vi "Boiler.vi"() -> ()   [LabVIEW 2025]
uses:
  Controls/Boiler Controls.ctl
  Controls/Boiler Simulation Controls.ctl
  Controls/Boiler Status Indicators.ctl
  Controls/States.ctl
panel:
  in  "stop":bool
  out "Boiler Status Indicators":T1 {"Time Count" format="%.2g"}
  in  "Boiler Simulation Controls":T2 {"Flame Sensor Value (%)" min=0.0 max=100.0 scale=0.0..100.0}
  in  "Boiler Controls":T3 {"Fuel Valve Position" min=0.0 max=100.0 scale=0.0..100.0 scale format="%.2f"}
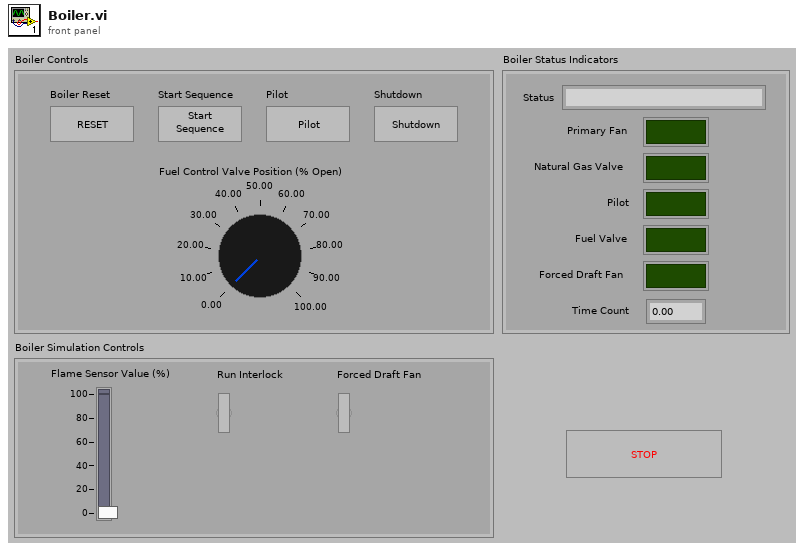
[diagram p1: front panel]
types:
  T1 = typedef "Boiler Status Indicators.ctl" = cluster{"Status":string, "Primary Fan":bool, "Natural Gas Valve":bool, "Pilot":bool, "Fuel Valve":bool, "Forced Draft Fan":bool, "Time Count":dbl}
  T2 = typedef "Boiler Simulation Controls.ctl" = cluster{"Flame Sensor Value (%)":dbl, "Run Interlock":bool, "Forced Draft Fan":bool}
  T3 = typedef "Boiler Controls.ctl" = cluster{"Boiler Reset":bool, "Start Sequence":bool, "Pilot":bool, "Shutdown":bool, "Fuel Valve Position":dbl}
  T4 = typedef "States.ctl" = enum16{"Initialization", "Lockout", "Ready", "Pre-Purge Start", "Pre-Purge Ongoing", "Pre-Purge Complete", "Wait Pilot", "Pilot-On", "Boiler Ready", "Fan On", "Boiler Running", "Shutdown Purge Start", "Shutdown Purge Ongoing", "Shutdown Purge Complete"}
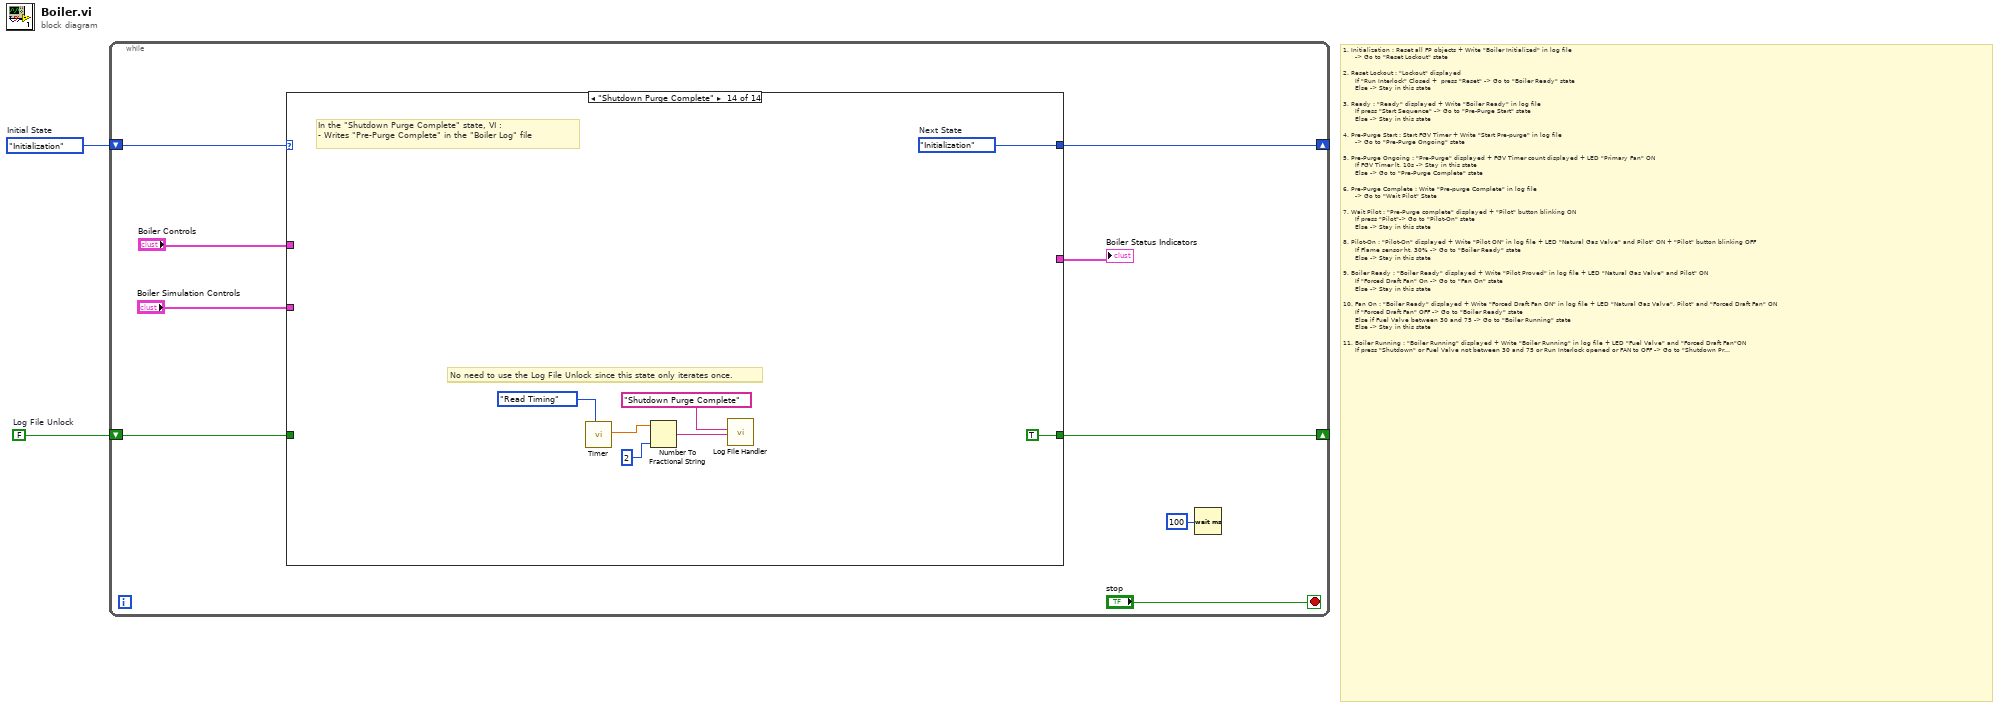
[diagram p0: block diagram]
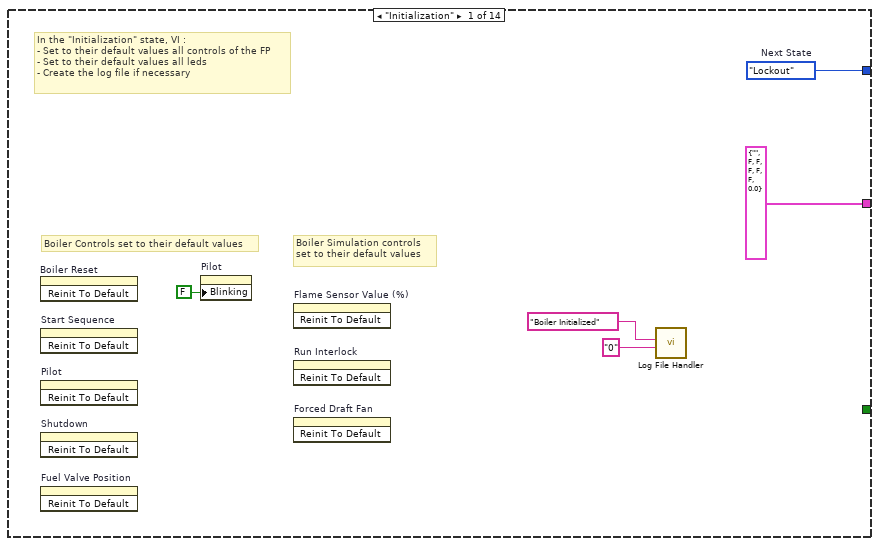
[diagram p2: hidden frame]
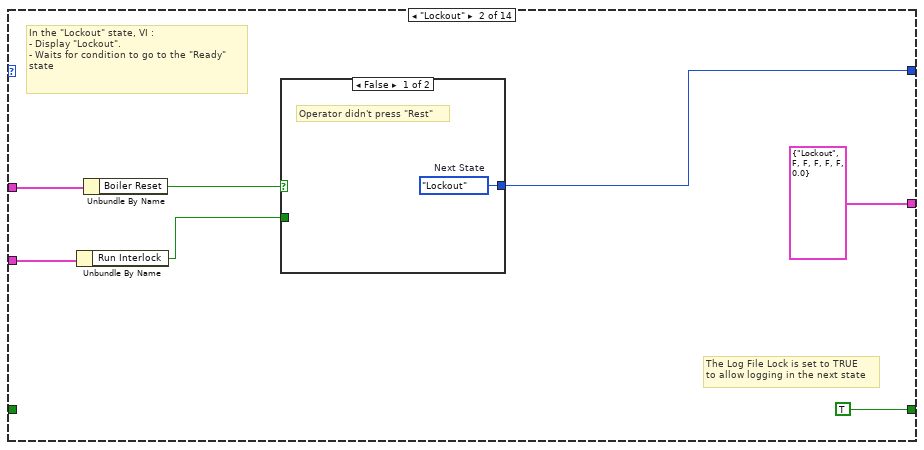
[diagram p3: hidden frame]
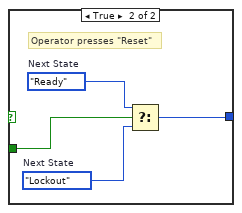
[diagram p4: hidden frame]
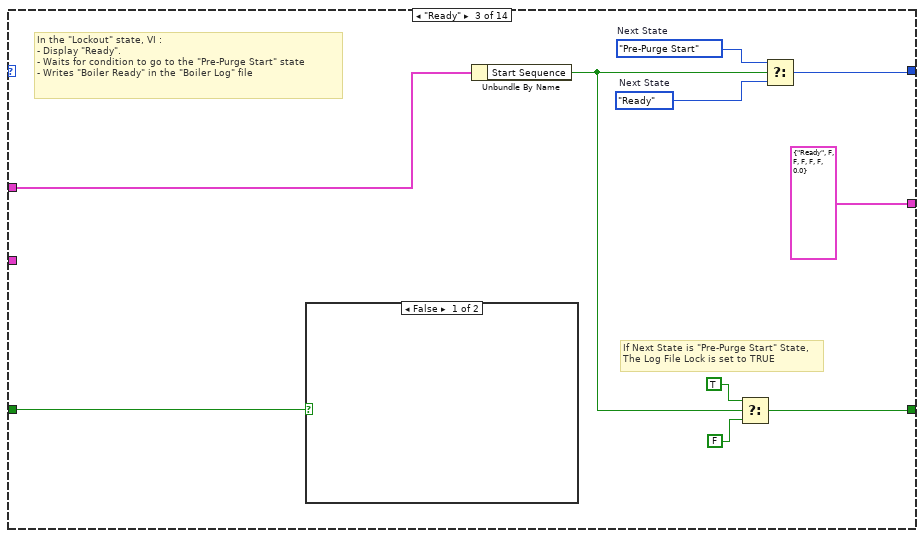
[diagram p5: hidden frame]
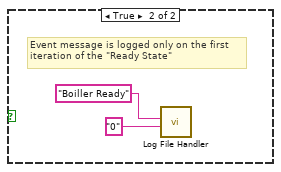
[diagram p6: hidden frame]
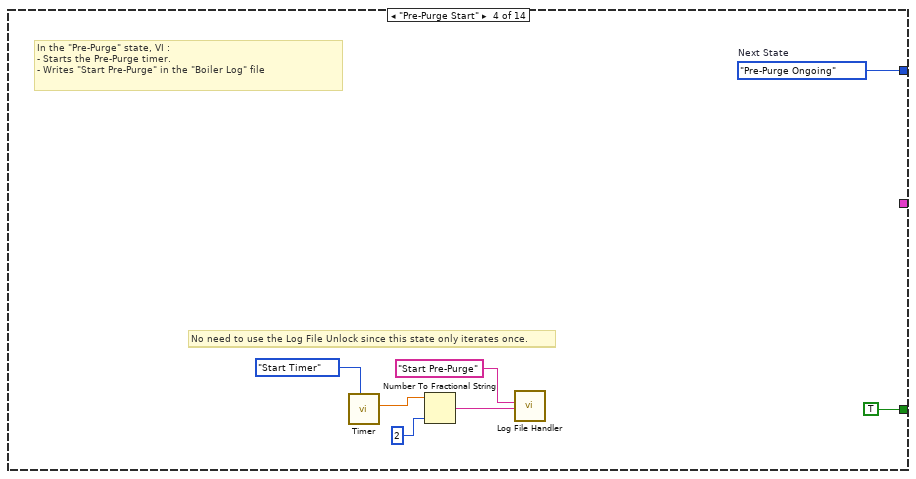
[diagram p7: hidden frame]
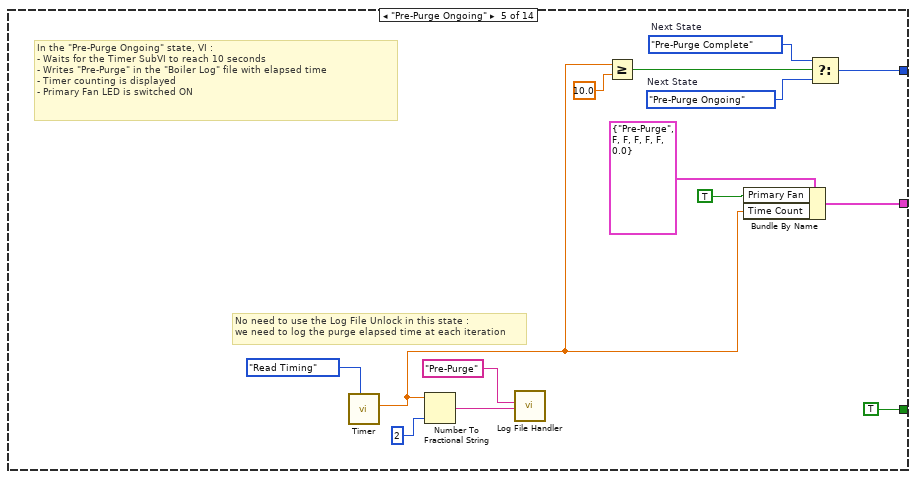
[diagram p8: hidden frame]
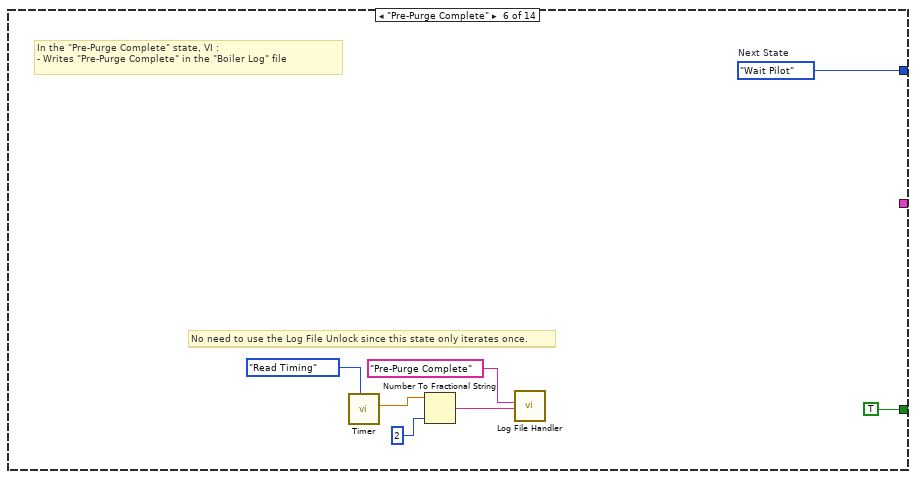
[diagram p9: hidden frame]
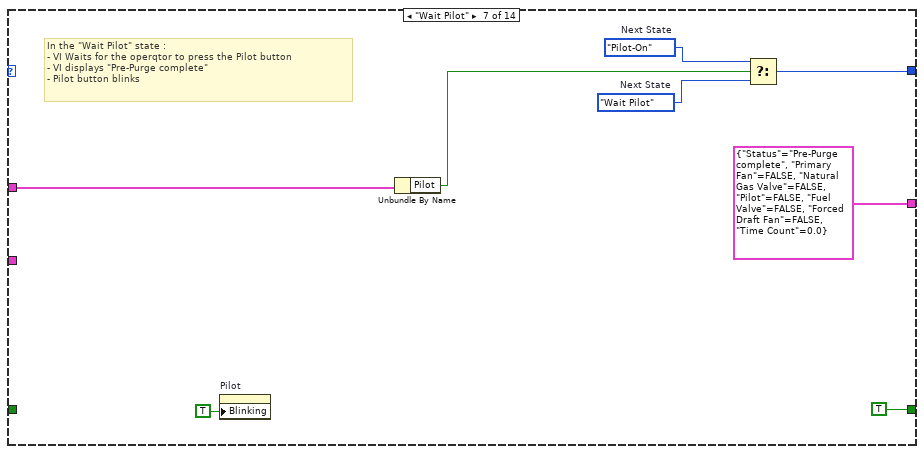
[diagram p10: hidden frame]
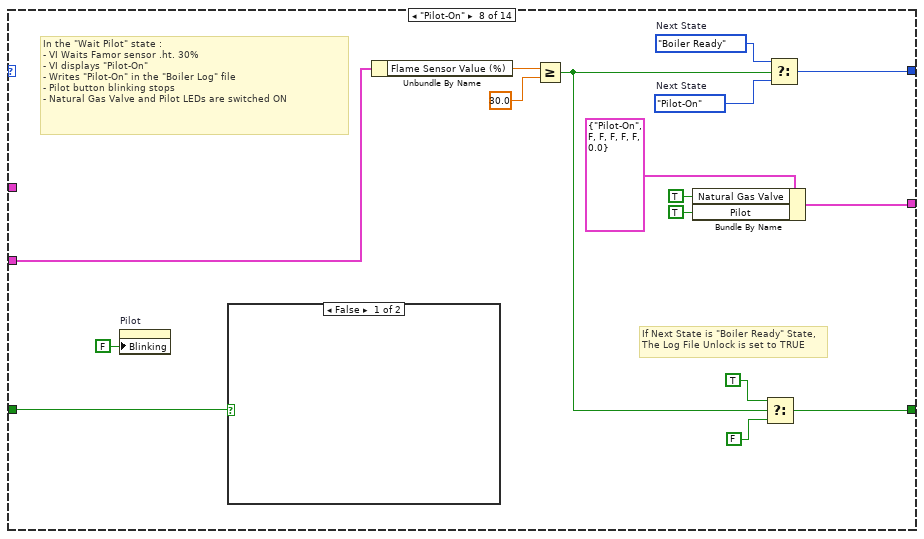
[diagram p11: hidden frame]
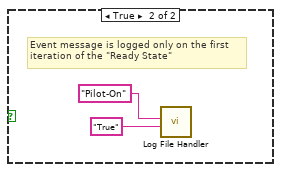
[diagram p12: hidden frame]
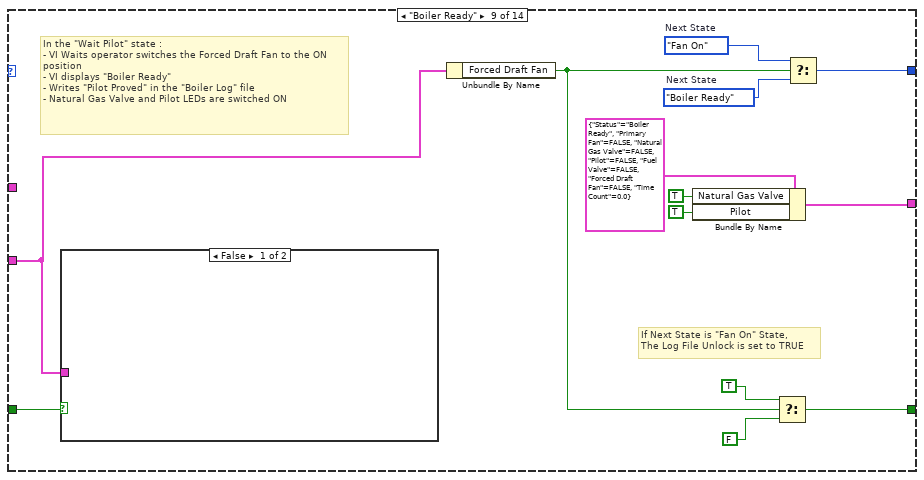
[diagram p13: hidden frame]
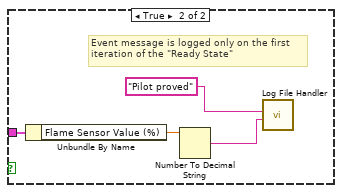
[diagram p14: hidden frame]
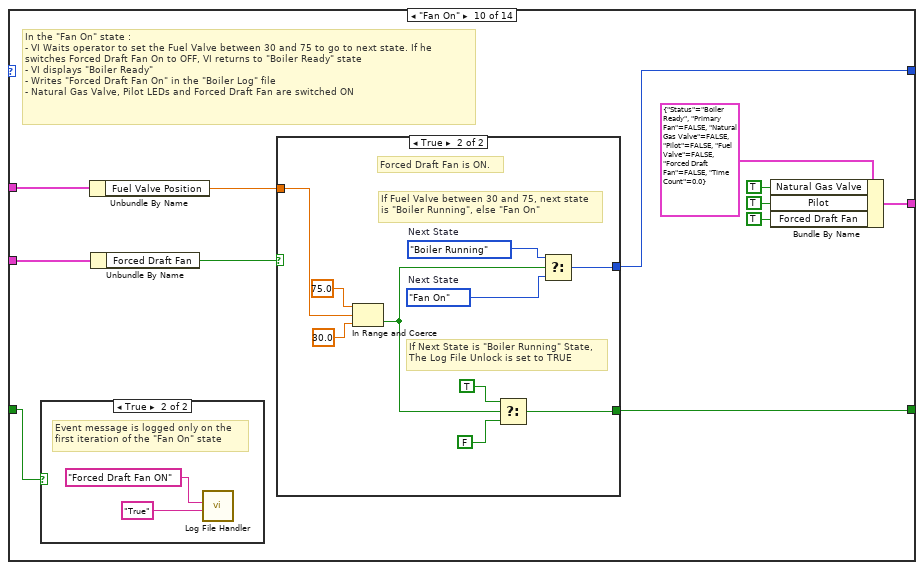
[diagram p15: hidden frame]
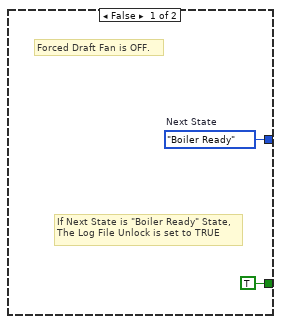
[diagram p16: hidden frame]
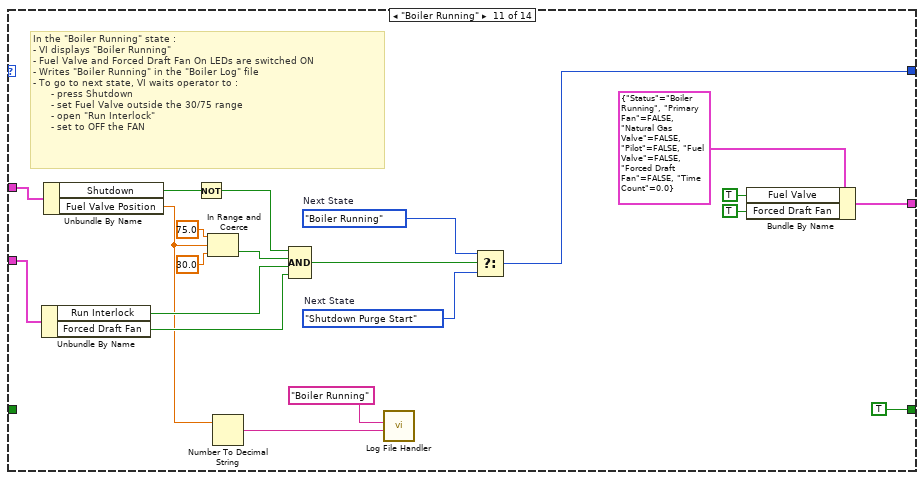
[diagram p18: hidden frame]
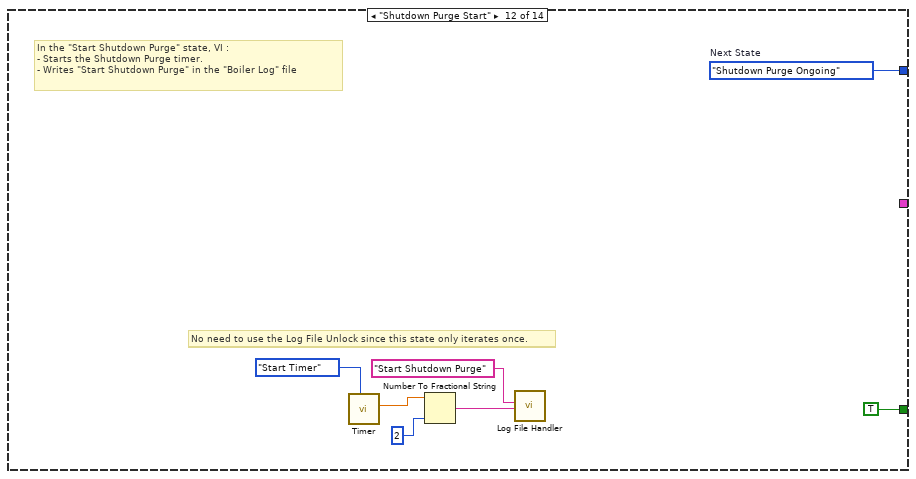
[diagram p19: hidden frame]
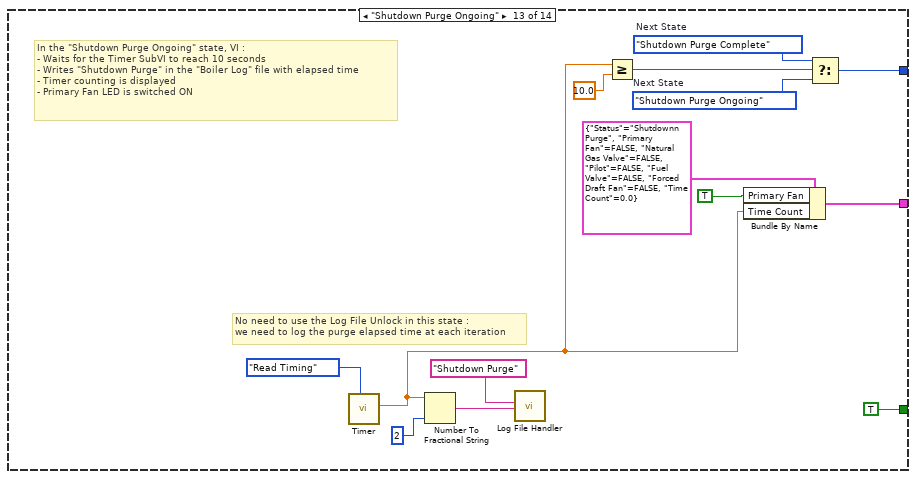
[diagram p20: hidden frame]
diagram:
  w1 = States."Initialization"  # Initial State
  w2 = FALSE  # Log File Unlock
  # "1. Initialization : Reset all FP objects + Write \"Boiler Initialized\" in log file\n      -> Go to \"Reset Lockout\" state\n\n2. Reset Lockout : \"Lockout\" displayed\n      If \"Run Interlock\" Closed +  press \"Reset\" -> Go to \"Boiler Ready\" state\n      Else -> Stay in this state\n\n3. Ready : \"Ready\" displayed + Write \"Boiler Ready\" in log file\n      If press \"Start Sequence\" -> Go to \"Pre-Purge Start\" state\n      Else -> Stay in this state\n\n4. Pre-Purge Start : Start FGV Timer + Write \"Start Pre-purge\" in log file\n      -> Go to \"Pre-Purge Ongoing\" state\n\n5. Pre-Purge Ongoing : \"Pre-Purge\" displayed + FGV Timer count displayed + LED \"Primary Fan\" ON\n      If FGV Timer lt. 10s -> Stay in this state\n      Else -> Go to \"Pre-Purge Complete\" state\n\n6. Pre-Purge Complete : Write \"Pre-purge Complete\" in log file\n      -> Go to \"Wait Pilot\" State \n\n7. Wait Pilot : \"Pre-Purge complete\" displayed + \"Pilot\" button blinking ON\n      If press \"Pilot\"-> Go to \"Pilot-On\" state\n      Else -> Stay in this state\n\n8. Pilot-On : \"Pilot-On\" displayed + Write \"Pilot ON\" in log file + LED \"Natural Gas Valve\" and Pilot\" ON + \"Pilot\" button blinking OFF\n      If Flame sensor ht. 30% -> Go to \"Boiler Ready\" state\n      Else -> Stay in this state\n\n9. Boiler Ready : \"Boiler Ready\" displayed + Write \"Pilot Proved\" in log file + LED \"Natural Gas Valve\" and Pilot\" ON\n      If \"Forced Draft Fan\" On -> Go to \"Fan On\" state\n      Else -> Stay in this state\n\n10. Fan On : \"Boiler Ready\" displayed + Write \"Forced Draft Fan ON\" in log file + LED \"Natural Gas Valve\", Pilot\" and \"Forced Draft Fan\" ON\n      If \"Forced Draft Fan\" OFF -> Go to \"Boiler Ready\" state\n      Else if Fuel Valve between 30 and 75 -> Go to \"Boiler Running\" state\n      Else -> Stay in this state\n\n11. Boiler Running : \"Boiler Running\" displayed + Write \"Boiler Running\" in log file + LED \"Fuel Valve\" and \"Forced Draft Fan\"ON\n      If press \"Shutdown\" or Fuel Valve not between 30 and 75 or Run Interlock opened or FAN to OFF -> Go to \"Shutdown Pre-Purge Start\" State\n      Else -> Stay in this state\n\n12. Shutdown Purge Start: : Start FGV Timer + Write \"Start Shutdown Purge\" in log file\n      -> Go to \"Shutdown Purge Ongoing\" state\n\n13. Shutdown Purge Ongoing : \"Purge\" displayed + FGV Timer count displayed + LED \"Primary Fan\" ON\n      If FGV Timer lt. 10s -> Stay in this state\n      Else -> Go to \"Shutdown Purge Complete\" state\n\n14. Shutdown Purge Complete : Write \"Shutdown purge Complete\" in log file\n      -> Go to \"Initilization\" State"
  n1 = while {
    shift-right: [w7] -> _
    shift-left: w2 -> [w8]
    shift-right: [w6] -> _
    shift-left: w1 -> [w5]
    stop <- "stop" stop-if-true
    n2 = case shown="\"Shutdown Purge Complete\"" w5 {
      tunnel: [T1 {"Status"="", "Primary Fan"=FALSE, "Natural Gas Valve"=FALSE, "Pilot"=FALSE, "Fuel Valve"=FALSE, "Forced Draft Fan"=FALSE, "Time Count"=0.0} ("Boiler Status Indicators") T1 {"Status"="Lockout", "Primary Fan"=FALSE, "Natural Gas Valve"=FALSE, "Pilot"=FALSE, "Fuel Valve"=FALSE, "Forced Draft Fan"=FALSE, "Time Count"=0.0} ("Boiler Status Indicators") T1 {"Status"="Ready", "Primary Fan"=FALSE, "Natural Gas Valve"=FALSE, "Pilot"=FALSE, "Fuel Valve"=FALSE, "Forced Draft Fan"=FALSE, "Time Count"=0.0} ("Boiler Status Indicators") _ w54 _ T1 {"Status"="Pre-Purge complete", "Primary Fan"=FALSE, "Natural Gas Valve"=FALSE, "Pilot"=FALSE, "Fuel Valve"=FALSE, "Forced Draft Fan"=FALSE, "Time Count"=0.0} ("Boiler Status Indicators") w87 w103 w118 w144 _ w172 _] -> w9
      tunnel: "Boiler Controls" -> [_ w22 w37 _ _ _ w74 _ _ w115 w158 _ _ _]
      tunnel: "Boiler Simulation Controls" -> [_ w21 _ _ _ _ _ w86 w102 w117 w155 _ _ _]
      tunnel: w8 -> [_ _ w34 _ _ _ _ w91 w107 w123 _ _ _ _]
      tunnel: [_ TRUE w30 TRUE TRUE TRUE TRUE w77 w95 w113 TRUE ("f") TRUE TRUE TRUE] -> w7
      tunnel: [w13 w17 w29 w41 w48 w62 w70 w81 w100 w112 w146 w159 w166 w180] -> w6
      frame "Initialization" {
        w13 = States."Lockout"  # Next State
        # "In the \"Initialization\" state, VI :\n- Set to their default values all controls of the FP\n- Set to their default values all leds\n- Create the log file if necessary"
        # "Boiler Simulation controls \nset to their default values"
        # "Boiler Controls set to their default values"
        n3 = invoke on="Boiler Reset" class="Bool" method="Reinit To Default"() -> ()  [unwired: 3 in, 3 out]
        n4 = invoke on="Start Sequence" class="Bool" method="Reinit To Default"() -> ()  [unwired: 3 in, 3 out]
        n5 = invoke on="Pilot" class="Bool" method="Reinit To Default"() -> ()  [unwired: 3 in, 3 out]
        n6 = invoke on="Shutdown" class="Bool" method="Reinit To Default"() -> ()  [unwired: 3 in, 3 out]
        n7 = invoke on="Fuel Valve Position" class="Knob (strict)" method="Reinit To Default"() -> ()  [unwired: 3 in, 3 out]
        n8 = property on="Pilot" class="Bool"("Blinking"=FALSE) -> ()  [unwired: 2 in, 2 out]
        n9 = invoke on="Flame Sensor Value (%)" class="Slide (strict)" method="Reinit To Default"() -> ()  [unwired: 3 in, 3 out]
        n10 = invoke on="Run Interlock" class="Bool (strict)" method="Reinit To Default"() -> ()  [unwired: 3 in, 3 out]
        n11 = invoke on="Forced Draft Fan" class="Bool (strict)" method="Reinit To Default"() -> ()  [unwired: 3 in, 3 out]
        n12 = call "Log File Handler.vi"("Event data"="0", "Event"="Boiler Initialized") -> ()  [unwired: 10 in]
      }
      frame "Lockout" {
        # "The Log File Lock is set to TRUE\nto allow logging in the next state"
        # "In the \"Lockout\" state, VI :\n- Display \"Lockout\".\n- Waits for condition to go to the \"Ready\" state"
        n13 = Unbundle By Name(w21) -> ("Run Interlock"=w19:bool)
        n14 = Unbundle By Name(w22) -> ("Boiler Reset"=w20:bool)
        n15 = case shown="False" w20 {
          tunnel: w19 -> [_ w28]
          tunnel: [w24 w25] -> w17
          frame False {
            w24 = States."Lockout"  # Next State
            # "Operator didn't press \"Rest\""
          }
          frame True {
            w26 = States."Lockout"  # Next State
            w27 = States."Ready"  # Next State
            # "Operator presses \"Reset\""
            n16 = Select(t=w27, s=w28, f=w26) -> (s? t:f=w25:T4)
          }
        }
      }
      frame "Ready" {
        w35 = States."Ready"  # Next State
        w36 = States."Pre-Purge Start"  # Next State
        # "In the \"Lockout\" state, VI :\n- Display \"Ready\".\n- Waits for condition to go to the \"Pre-Purge Start\" state\n- Writes \"Boiler Ready\" in the \"Boiler Log\" file"
        # "If Next State is \"Pre-Purge Start\" State,\nThe Log File Lock is set to TRUE"
        n17 = case shown="False" w34 {
          frame False {
          }
          frame True {
            # "Event message is logged only on the first\niteration of the \"Ready State\""
            n18 = call "Log File Handler.vi"("Event data"="0", "Event"="Boiller Ready") -> ()  [unwired: 10 in]
          }
        }
        n19 = Unbundle By Name(w37) -> ("Start Sequence"=w33:bool)
        n20 = Select(t=TRUE, s=w33, f=FALSE) -> (s? t:f=w30:bool)
        n21 = Select(t=w36, s=w33, f=w35) -> (s? t:f=w29:T4)
      }
      frame "Pre-Purge Start" {
        w41 = States."Pre-Purge Ongoing"  # Next State
        # "No need to use the Log File Unlock since this state only iterates once."
        # "No need to use the Log File Unlock since this state only iterates once."
        # "In the \"Pre-Purge\" state, VI :\n- Starts the Pre-Purge timer.\n- Writes \"Start Pre-Purge\" in the \"Boiler Log\" file"
        n22 = call "Timer.vi"("Operation"=enum16{"Start Timer", "Read Timing"}."Start Timer") -> ("Elapsed time"=w46:dbl)  [unwired: 10 in]
        n23 = Number To Fractional String(number=w46, precision (6)=i16 2) -> (F-format string=w45:string)  [unwired: 2 in]
        n24 = call "Log File Handler.vi"("Event data"=w45, "Event"="Start Pre-Purge") -> ()  [unwired: 10 in]
      }
      frame "Pre-Purge Ongoing" {
        w49 = States."Pre-Purge Complete"  # Next State
        w50 = States."Pre-Purge Ongoing"  # Next State
        # "No need to use the Log File Unlock in this state : \nwe need to log the purge elapsed time at each iteration"
        # "In the \"Pre-Purge Ongoing\" state, VI :\n- Waits for the Timer SubVI to reach 10 seconds \n- Writes \"Pre-Purge\" in the \"Boiler Log\" file with elapsed time\n- Timer counting is displayed \n- Primary Fan LED is switched ON"
        n25 = call "Timer.vi"("Operation"=enum16{"Start Timer", "Read Timing"}."Read Timing") -> ("Elapsed time"=w53:dbl)  [unwired: 10 in]
        n26 = Number To Fractional String(number=w53, precision (6)=i16 2) -> (F-format string=w60:string)  [unwired: 2 in]
        n27 = call "Log File Handler.vi"("Event data"=w60, "Event"="Pre-Purge") -> ()  [unwired: 10 in]
        n28 = Greater Or Equal?(x=w53, y=10.0) -> (x >= y?=w51:bool)
        n29 = Bundle By Name(cluster=T1 {"Status"="Pre-Purge", "Primary Fan"=FALSE, "Natural Gas Valve"=FALSE, "Pilot"=FALSE, "Fuel Valve"=FALSE, "Forced Draft Fan"=FALSE, "Time Count"=0.0} ("Boiler Status Indicators"), "Primary Fan"=TRUE, "Time Count"=w53) -> (w54:T1)
        n30 = Select(t=w49, s=w51, f=w50) -> (s? t:f=w48:T4)
      }
      frame "Pre-Purge Complete" {
        w62 = States."Wait Pilot"  # Next State
        # "No need to use the Log File Unlock since this state only iterates once."
        # "No need to use the Log File Unlock since this state only iterates once."
        # "In the \"Pre-Purge Complete\" state, VI :\n- Writes \"Pre-Purge Complete\" in the \"Boiler Log\" file"
        n31 = call "Timer.vi"("Operation"=enum16{"Start Timer", "Read Timing"}."Read Timing") -> ("Elapsed time"=w67:dbl)  [unwired: 10 in]
        n32 = Number To Fractional String(number=w67, precision (6)=i16 2) -> (F-format string=w66:string)  [unwired: 2 in]
        n33 = call "Log File Handler.vi"("Event data"=w66, "Event"="Pre-Purge Complete") -> ()  [unwired: 10 in]
      }
      frame "Wait Pilot" {
        w71 = States."Wait Pilot"  # Next State
        w72 = States."Pilot-On"  # Next State
        # "In the \"Wait Pilot\" state : \n- VI Waits for the operqtor to press the Pilot button \n- VI displays \"Pre-Purge complete\"\n- Pilot button blinks"
        n34 = property on="Pilot" class="Bool"("Blinking"=TRUE) -> ()  [unwired: 2 in, 2 out]
        n35 = Unbundle By Name(w74) -> ("Pilot"=w73:bool)
        n36 = Select(t=w72, s=w73, f=w71) -> (s? t:f=w70:T4)
      }
      frame "Pilot-On" {
        w82 = States."Pilot-On"  # Next State
        w83 = States."Boiler Ready"  # Next State
        # "If Next State is \"Boiler Ready\" State,\nThe Log File Unlock is set to TRUE"
        # "In the \"Wait Pilot\" state : \n- VI Waits Famor sensor .ht. 30% \n- VI displays \"Pilot-On\"\n- Writes \"Pilot-On\" in the \"Boiler Log\" file\n- Pilot button blinking stops\n- Natural Gas Valve and Pilot LEDs are switched ON"
        n37 = property on="Pilot" class="Bool"("Blinking"=FALSE) -> ()  [unwired: 2 in, 2 out]
        n38 = case shown="False" w91 {
          frame False {
          }
          frame True {
            # "Event message is logged only on the first\niteration of the \"Ready State\""
            n39 = call "Log File Handler.vi"("Event data"="True", "Event"="Pilot-On") -> ()  [unwired: 10 in]
          }
        }
        n40 = Unbundle By Name(w86) -> ("Flame Sensor Value (%)"=w85:dbl)
        n41 = Greater Or Equal?(x=w85, y=30.0) -> (x >= y?=w80:bool)
        n42 = Bundle By Name(cluster=T1 {"Status"="Pilot-On", "Primary Fan"=FALSE, "Natural Gas Valve"=FALSE, "Pilot"=FALSE, "Fuel Valve"=FALSE, "Forced Draft Fan"=FALSE, "Time Count"=0.0} ("Boiler Status Indicators"), "Natural Gas Valve"=TRUE, "Pilot"=TRUE) -> (w87:T1)
        n43 = Select(t=TRUE, s=w80, f=FALSE) -> (s? t:f=w77:bool)
        n44 = Select(t=w83, s=w80, f=w82) -> (s? t:f=w81:T4)
      }
      frame "Boiler Ready" {
        w99 = States."Boiler Ready"  # Next State
        w101 = States."Fan On"  # Next State
        # "If Next State is \"Fan On\" State,\nThe Log File Unlock is set to TRUE"
        # "In the \"Wait Pilot\" state : \n- VI Waits operator switches the Forced Draft Fan to the ON position\n- VI displays \"Boiler Ready\"\n- Writes \"Pilot Proved\" in the \"Boiler Log\" file\n- Natural Gas Valve and Pilot LEDs are switched ON"
        n45 = case shown="False" w107 {
          tunnel: w102 -> [_ w110]
          frame False {
          }
          frame True {
            # "Event message is logged only on the first\niteration of the \"Ready State\""
            n46 = Unbundle By Name(w110) -> ("Flame Sensor Value (%)"=w109:dbl)
            n47 = Number To Decimal String(number=w109) -> (decimal integer string=w108:string)  [unwired: 1 in]
            n48 = call "Log File Handler.vi"("Event data"=w108, "Event"="Pilot proved") -> ()  [unwired: 10 in]
          }
        }
        n49 = Unbundle By Name(w102) -> ("Forced Draft Fan"=w98:bool)
        n50 = Bundle By Name(cluster=T1 {"Status"="Boiler Ready", "Primary Fan"=FALSE, "Natural Gas Valve"=FALSE, "Pilot"=FALSE, "Fuel Valve"=FALSE, "Forced Draft Fan"=FALSE, "Time Count"=0.0} ("Boiler Status Indicators"), "Natural Gas Valve"=TRUE, "Pilot"=TRUE) -> (w103:T1)
        n51 = Select(t=TRUE, s=w98, f=FALSE) -> (s? t:f=w95:bool)
        n52 = Select(t=w101, s=w98, f=w99) -> (s? t:f=w100:T4)
      }
      frame "Fan On" {
        # "In the \"Fan On\" state : \n- VI Waits operator to set the Fuel Valve between 30 and 75 to go to next state. If he switches Forced Draft Fan On to OFF, VI returns to \"Boiler Ready\" state\n- VI displays \"Boiler Ready\"\n- Writes \"Forced Draft Fan On\" in the \"Boiler Log\" file\n- Natural Gas Valve, Pilot LEDs and Forced Draft Fan are switched ON"
        n53 = case shown="True" w123 {
          frame False {
          }
          frame True {
            # "Event message is logged only on the\nfirst iteration of the \"Fan On\" state"
            n54 = call "Log File Handler.vi"("Event data"="True", "Event"="Forced Draft Fan ON") -> ()  [unwired: 10 in]
          }
        }
        n55 = Unbundle By Name(w115) -> ("Fuel Valve Position"=w114:dbl)
        n56 = Unbundle By Name(w117) -> ("Forced Draft Fan"=w116:bool)
        n57 = case shown="True" w116 {
          tunnel: w114 -> [_ w135]
          tunnel: [TRUE ("f") w127] -> w113
          tunnel: [w125 w126] -> w112
          frame False {
            w125 = States."Boiler Ready"  # Next State
            # "If Next State is \"Boiler Ready\" State,\nThe Log File Unlock is set to TRUE"
            # "Forced Draft Fan is OFF."
          }
          frame True {
            w130 = States."Fan On"  # Next State
            w131 = States."Boiler Running"  # Next State
            # "If Next State is \"Boiler Running\" State,\nThe Log File Unlock is set to TRUE"
            # "If Fuel Valve between 30 and 75, next state\nis \"Boiler Running\", else \"Fan On\""
            # "Forced Draft Fan is ON."
            n58 = In Range and Coerce(upper limit=75.0, x=w135, lower limit=30.0) -> (In Range?=w132:bool)  [unwired: 1 out]
            n59 = Select(t=TRUE, s=w132, f=FALSE) -> (s? t:f=w127:bool)
            n60 = Select(t=w131, s=w132, f=w130) -> (s? t:f=w126:T4)
          }
        }
        n61 = Bundle By Name(cluster=T1 {"Status"="Boiler Ready", "Primary Fan"=FALSE, "Natural Gas Valve"=FALSE, "Pilot"=FALSE, "Fuel Valve"=FALSE, "Forced Draft Fan"=FALSE, "Time Count"=0.0} ("Boiler Status Indicators"), "Natural Gas Valve"=TRUE, "Pilot"=TRUE, "Forced Draft Fan"=TRUE) -> (w118:T1)
      }
      frame "Boiler Running" {
        w147 = States."Shutdown Purge Start"  # Next State
        w148 = States."Boiler Running"  # Next State
        # "In the \"Boiler Running\" state : \n- VI displays \"Boiler Running\"\n- Fuel Valve and Forced Draft Fan On LEDs are switched ON\n- Writes \"Boiler Running\" in the \"Boiler Log\" file\n- To go to next state, VI waits operator to :\n      - press Shutdown\n      - set Fuel Valve outside the 30/75 range\n      - open \"Run Interlock\"\n      - set to OFF the FAN"
        n62 = Unbundle By Name(w155) -> ("Run Interlock"=w151:bool, "Forced Draft Fan"=w150:bool)
        n63 = Unbundle By Name(w158) -> ("Shutdown"=w154:bool, "Fuel Valve Position"=w140:dbl)
        n64 = Not(x=w154) -> (.not. x?=w153:bool)
        n65 = In Range and Coerce(upper limit=75.0, x=w140, lower limit=30.0) -> (In Range?=w152:bool)  [unwired: 1 out]
        n66 = Number To Decimal String(number=w140) -> (decimal integer string=w139:string)  [unwired: 1 in]
        n67 = Compound Arithmetic op=AND(w153, w152, w151, w150) -> (w149:bool)
        n68 = call "Log File Handler.vi"("Event data"=w139, "Event"="Boiler Running") -> ()  [unwired: 10 in]
        n69 = Select(t=w148, s=w149, f=w147) -> (s? t:f=w146:T4)
        n70 = Bundle By Name(cluster=T1 {"Status"="Boiler Running", "Primary Fan"=FALSE, "Natural Gas Valve"=FALSE, "Pilot"=FALSE, "Fuel Valve"=FALSE, "Forced Draft Fan"=FALSE, "Time Count"=0.0} ("Boiler Status Indicators"), "Fuel Valve"=TRUE, "Forced Draft Fan"=TRUE) -> (w144:T1)
      }
      frame "Shutdown Purge Start" {
        w159 = States."Shutdown Purge Ongoing"  # Next State
        # "No need to use the Log File Unlock since this state only iterates once."
        # "No need to use the Log File Unlock since this state only iterates once."
        # "In the \"Start Shutdown Purge\" state, VI :\n- Starts the Shutdown Purge timer.\n- Writes \"Start Shutdown Purge\" in the \"Boiler Log\" file"
        n71 = call "Timer.vi"("Operation"=enum16{"Start Timer", "Read Timing"}."Start Timer") -> ("Elapsed time"=w164:dbl)  [unwired: 10 in]
        n72 = Number To Fractional String(number=w164, precision (6)=i16 2) -> (F-format string=w163:string)  [unwired: 2 in]
        n73 = call "Log File Handler.vi"("Event data"=w163, "Event"="Start Shutdown Purge") -> ()  [unwired: 10 in]
      }
      frame "Shutdown Purge Ongoing" {
        w167 = States."Shutdown Purge Complete"  # Next State
        w168 = States."Shutdown Purge Ongoing"  # Next State
        # "No need to use the Log File Unlock in this state : \nwe need to log the purge elapsed time at each iteration"
        # "In the \"Shutdown Purge Ongoing\" state, VI :\n- Waits for the Timer SubVI to reach 10 seconds \n- Writes \"Shutdown Purge\" in the \"Boiler Log\" file with elapsed time\n- Timer counting is displayed \n- Primary Fan LED is switched ON"
        n74 = call "Timer.vi"("Operation"=enum16{"Start Timer", "Read Timing"}."Read Timing") -> ("Elapsed time"=w171:dbl)  [unwired: 10 in]
        n75 = Number To Fractional String(number=w171, precision (6)=i16 2) -> (F-format string=w178:string)  [unwired: 2 in]
        n76 = call "Log File Handler.vi"("Event data"=w178, "Event"="Shutdown Purge") -> ()  [unwired: 10 in]
        n77 = Greater Or Equal?(x=w171, y=10.0) -> (x >= y?=w169:bool)
        n78 = Bundle By Name(cluster=T1 {"Status"="Shutdownn Purge", "Primary Fan"=FALSE, "Natural Gas Valve"=FALSE, "Pilot"=FALSE, "Fuel Valve"=FALSE, "Forced Draft Fan"=FALSE, "Time Count"=0.0} ("Boiler Status Indicators"), "Primary Fan"=TRUE, "Time Count"=w171) -> (w172:T1)
        n79 = Select(t=w167, s=w169, f=w168) -> (s? t:f=w166:T4)
      }
      frame "Shutdown Purge Complete" {
        w180 = States."Initialization"  # Next State
        # "No need to use the Log File Unlock since this state only iterates once."
        # "No need to use the Log File Unlock since this state only iterates once."
        # "In the \"Shutdown Purge Complete\" state, VI :\n- Writes \"Pre-Purge Complete\" in the \"Boiler Log\" file"
        n80 = call "Timer.vi"("Operation"=enum16{"Start Timer", "Read Timing"}."Read Timing") -> ("Elapsed time"=w185:dbl)  [unwired: 10 in]
        n81 = Number To Fractional String(number=w185, precision (6)=i16 2) -> (F-format string=w184:string)  [unwired: 2 in]
        n82 = call "Log File Handler.vi"("Event data"=w184, "Event"="Shutdown Purge Complete") -> ()  [unwired: 10 in]
      }
    }
    "Boiler Status Indicators" <- w9
    n83 = Wait (ms)(milliseconds to wait=u32 100) -> ()  [unwired: 1 out]
  }
